vi "Get Process info.vi"(8 "error in (no error)":errorcluster, 11 "processName":string) -> (0 "error out":errorcluster, 1 "Peak VirtualMem Size":i64, 2 "VirtualMem Size":i64, 3 "Total CPU Seconds":dbl, 4 "StartTime":timestamp)   [LabVIEW 2020, in "Collector.lvlib" / "Process Collector.lvclass"]
uses:
  Process Collector.lvclass
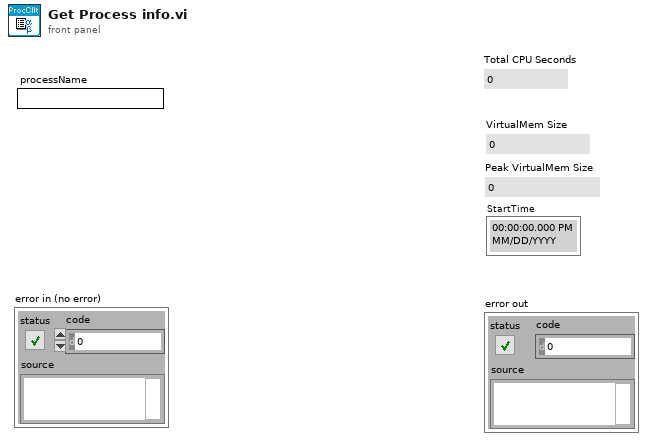
[diagram p1: front panel]
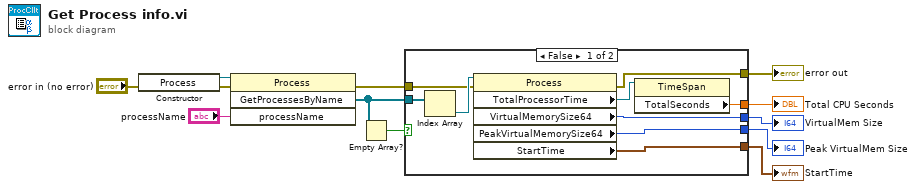
[diagram p0: block diagram]
diagram:
  n1 = constructor class="Process"(error in="error in (no error)") -> (reference out=w12:refnum<k24>, error out=w11:errorcluster)  [unwired: 2 in, 1 out]
  n2 = invoke class="Process" method="GetProcessesByName"(reference=w12, error in=w11, "processName"="processName") -> (error out=w4:errorcluster, "GetProcessesByName"=w3:refnum<k24>[])  [unwired: 1 in, 2 out]
  n3 = Empty Array?(array=w3) -> (empty?=w2:bool)
  n4 = case shown="False" w2 {
    tunnel: [w20 _] -> w10
    tunnel: [w19 _] -> w9
    tunnel: [w18 _] -> w8
    tunnel: [w16 _] -> w7
    tunnel: w4 -> [w15 w22]
    tunnel: w3 -> [w14 _]
    tunnel: [w13 w22] -> w1
    frame False {
      n5 = Index Array(array=w14) -> (element=w21:refnum<k24>)  [unwired: 1 in]
      n6 = property class="Process"(reference=w21, error in=w15) -> (error out=w13:errorcluster, "TotalProcessorTime"=w17:refnum<k24>, "VirtualMemorySize64"=w20:i64, "PeakVirtualMemorySize64"=w19:i64, "StartTime"=w18:timestamp)  [unwired: 1 out]
      n7 = property class="TimeSpan"(reference=w17) -> ("TotalSeconds"=w16:dbl)  [unwired: 1 in, 2 out]
    }
    frame True {
    }
  }
  "VirtualMem Size" <- w10
  "Peak VirtualMem Size" <- w9
  "StartTime" <- w8
  "Total CPU Seconds" <- w7
  "error out" <- w1
